vi "Matrix_Fill.vi"(9 "Value":dbl, 11 "input matrix":T1) -> (3 "output matrix":T1)   [LabVIEW 2019, in "Trajectory_Library.lvlib"]
doc: "Creates a new LINEAR SYSTEM data cluster with the specified values. \n\n\nInputs: \n - XXX -- XXX.\n\nOutputs:\n - XXX -- XXX."
uses:
  <vilib>/Analysis/Matrix/Datatypes/RealMatrix.ctl
  Trajectory_Library.lvlib
  <vilib>/Analysis/Matrix/NI_Matrix.lvlib
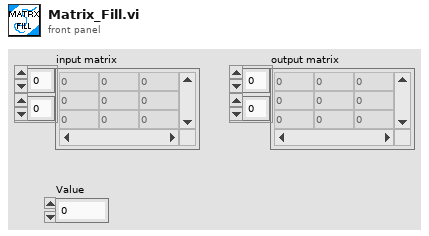
[diagram p1: front panel]
types:
  T1 = typedef "NI_Matrix.lvlib/RealMatrix.ctl" = dbl[][]
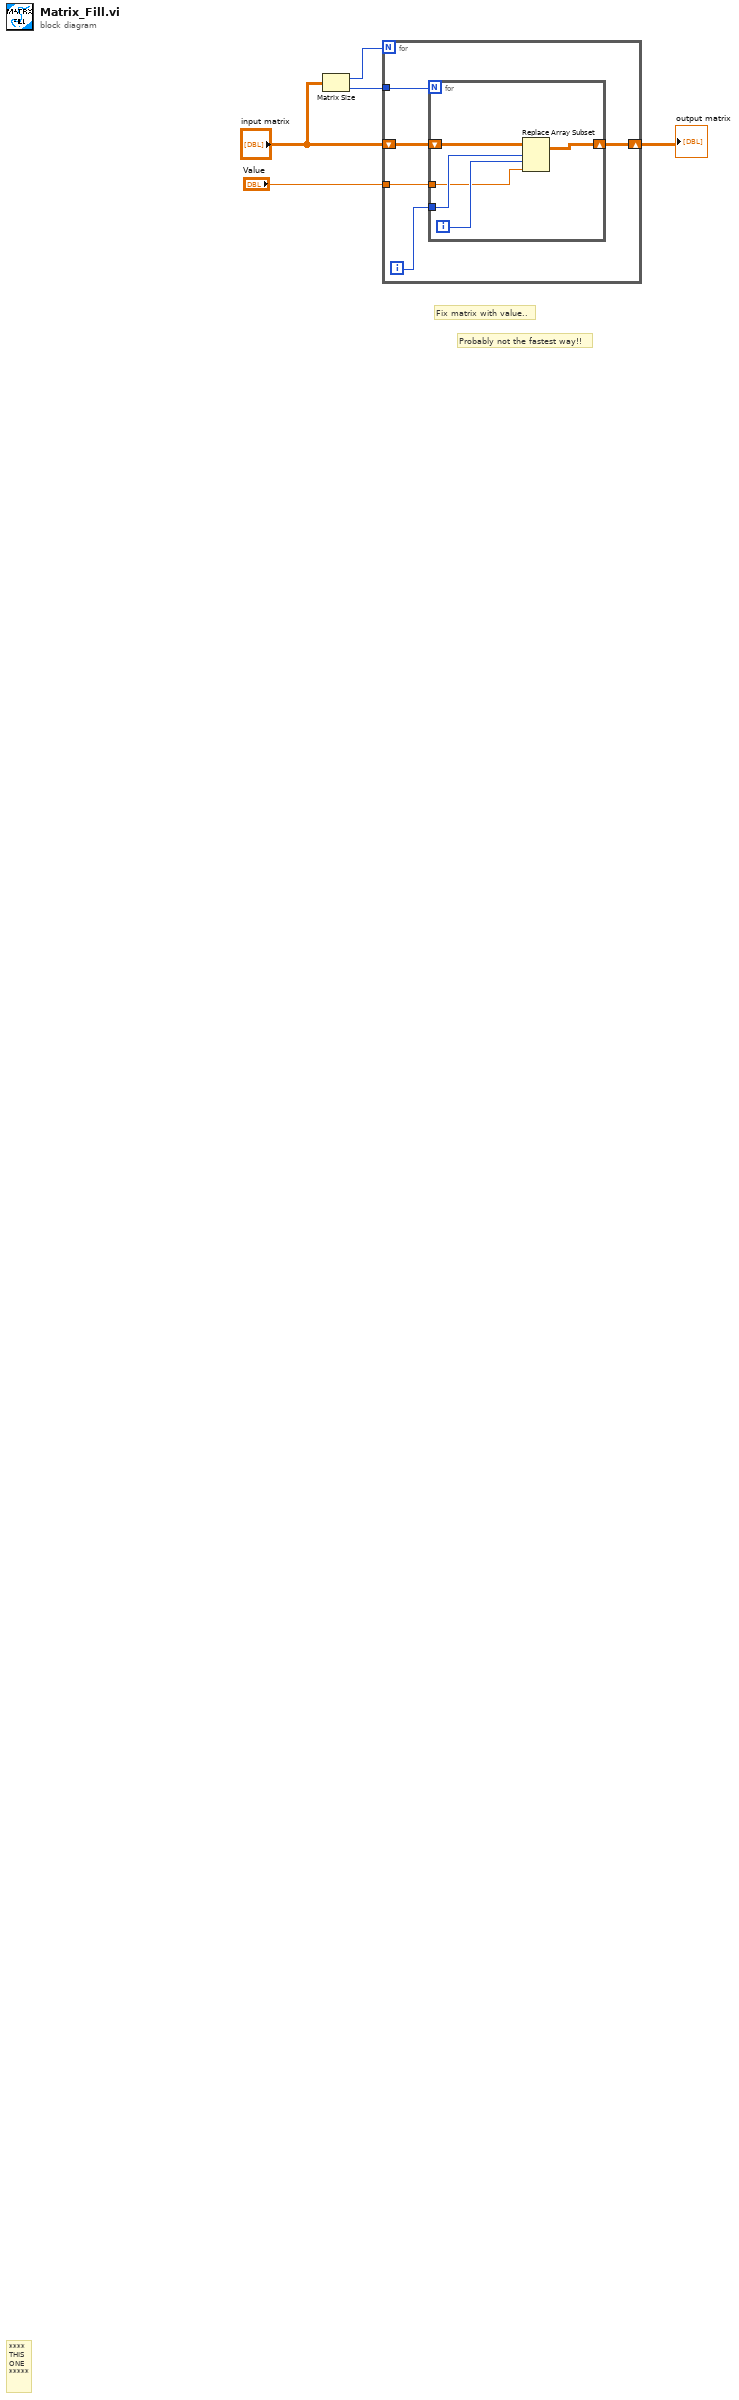
[diagram p0: block diagram]
diagram:
  # "Probably not the fastest way!!"
  # "Fix matrix with value.."
  # "****\nTHIS\nONE\n*****"
  n1 = Matrix Size(0:"input matrix") -> (1:w4:i32, 2:w3:i32)
  n2 = for {
    N: w4 -> [_]
    shift-right: [w7] -> w2
    shift-left: "input matrix" -> [w10]
    tunnel: w3 -> [w8]
    tunnel: "Value" -> [w6]
    i -> [w9]
    n3 = for {
      N: w8 -> [_]
      shift-right: [w12] -> w7
      shift-left: w10 -> [w15]
      tunnel: w9 -> [w13]
      tunnel: w6 -> [w11]
      i -> [w14]
      n4 = Replace Array Subset(array=w15, new element=w11, index (row)=w13, index (col)=w14) -> (w12:T1)
    }
  }
  "output matrix" <- w2
